vi "CreateEventsDialog.vi"(8 "error in (no error)":errorcluster, 11 "DQMH_Modules":refnum<class "DQMHModuleNode.lvclass">[](array[class])) -> (0 "error out":errorcluster)   [LabVIEW 2020, in "DqmhModuleDiagramGraph.lvclass"]
uses:
  <resource>/Framework/Providers/Open_GDS/UML/DqmhModuleDiagramGraph_class/DqmhModuleDiagramGraph.lvclass
  <resource>/Framework/Providers/Open_GDS/UML/DQMHModuleNode_class/DQMHModuleNode.lvclass
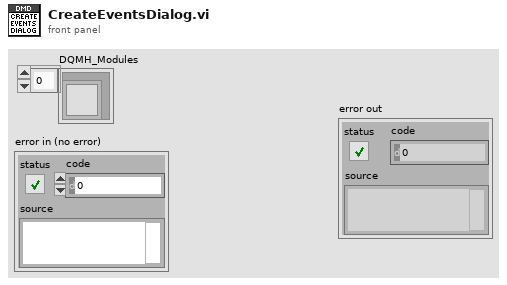
[diagram p1: front panel]
types:
  T1 = enum16{"Request", "Broadcast", "Request and Wait for Reply", "Round Trip"}
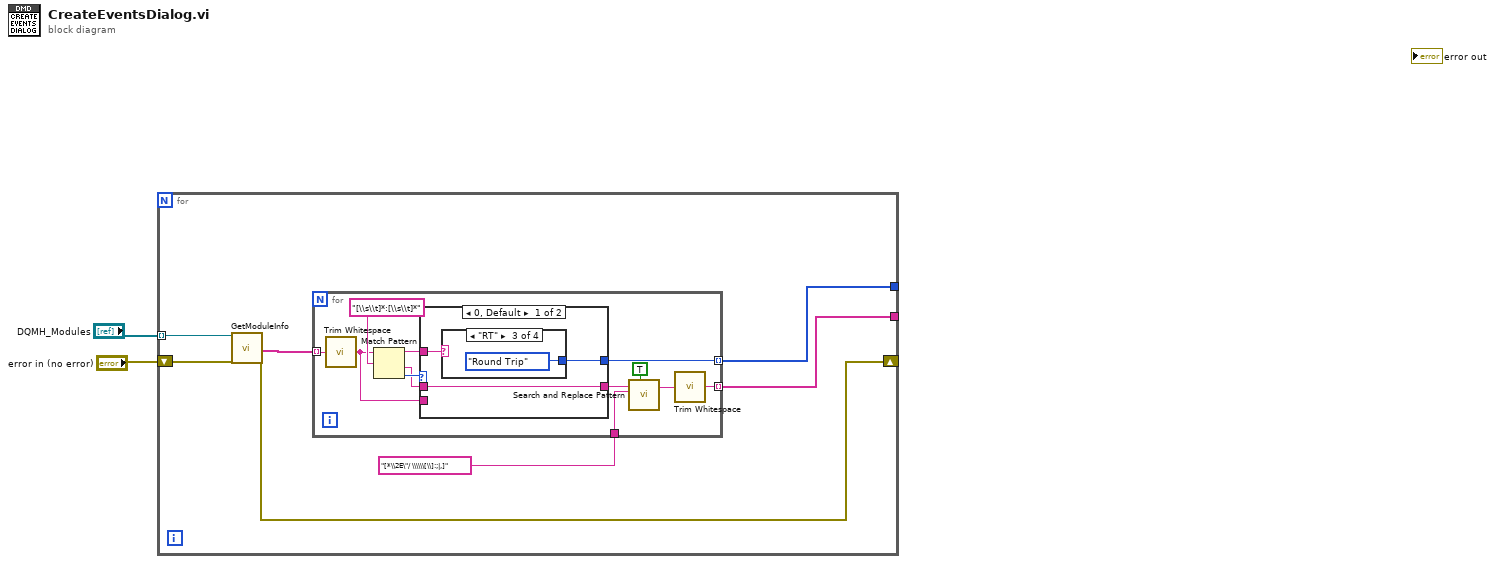
[diagram p0: block diagram]
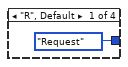
[diagram p2: hidden frame]
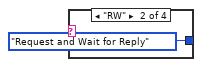
[diagram p3: hidden frame]
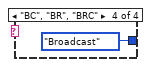
[diagram p4: hidden frame]
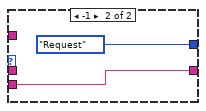
[diagram p5: hidden frame]
diagram:
  n1 = for {
    tunnel: [w7] -> _
    tunnel: [w6] -> _
    tunnel: "DQMH_Modules" -> [w5] mode=indexing
    shift-right: [w3] -> _
    shift-left: "error in (no error)" -> [w4]
    n2 = call-dynamic "GetModuleInfo.vi"("reference in"=w5, "error in (no error)"=w4) -> ("Events"=w9:string[], "error out"=w3:errorcluster)  [unwired: 6 in, 10 out]
    n3 = for {
      tunnel: w9 -> [w21] mode=indexing
      tunnel: [w10] -> w6 mode=indexing
      tunnel: [w18] -> w7 mode=indexing
      tunnel: "[*\\2E\"/ \\\\\\[\\]:;|,]" ("regular expression") -> [w11]
      n4 = call <vilib>:"Trim Whitespace.vi"("string"=w21) -> ("trimmed string"=w15:string)  [unwired: 1 in]
      n5 = Match Pattern(string=w15, regular expression="[\\s\\t]*:[\\s\\t]*") -> (before substring=w17:string, after substring=w16:string, offset past match=w19:i32)  [unwired: 1 in, 1 out]
      n6 = case shown="0, Default" w19 {
        tunnel: w16 -> [w22 _]
        tunnel: [w22 w29] -> w14
        tunnel: [w23 T1."Request" ("Event Type")] -> w18
        tunnel: w17 -> [w24 _]
        tunnel: w15 -> [_ w29]
        frame 0, Default {
          n7 = case shown="\"RT\"" w24 {
            tunnel: [T1."Request" ("Event Type") T1."Request and Wait for Reply" ("Event Type") T1."Round Trip" ("Event Type") T1."Broadcast" ("Event Type")] -> w23
            frame "R", Default {
            }
            frame "RW" {
            }
            frame "RT" {
            }
            frame "BC", "BR", "BRC" {
            }
          }
        }
        frame -1 {
        }
      }
      n8 = call <vilib>:"Search and Replace Pattern.vi"("string"=w14, "regular expression (\"\")"=w11, "replace all? (F)"=TRUE) -> ("result string"=w13:string)  [unwired: 2 in, 1 out]
      n9 = call <vilib>:"Trim Whitespace.vi"("string"=w13) -> ("trimmed string"=w10:string)  [unwired: 1 in]
    }
  }
